vi "Read Private Stop.vi"(11 "Base UI Actor in":refnum<class "Base UI Actor.lvclass">) -> (2 "Private Stop":refnum<user-event>)   [LabVIEW 2016, in "Base UI Actor.lvlib" / "Base UI Actor.lvclass"]
uses:
  Base UI Actor.lvclass
  Base UI Actor.lvclass/Base UI Actor.ctl
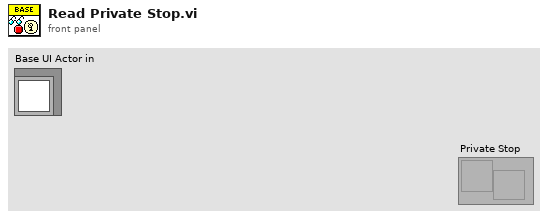
[diagram p1: front panel]
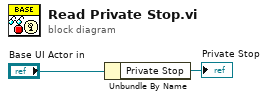
[diagram p0: block diagram]
diagram:
  n1 = Unbundle By Name("Base UI Actor in") -> ("Private Stop"=→"Private Stop":refnum<user-event>)
